vi "Build copy.vi"() -> ()   [LabVIEW 2017]
panel:
  out "Boolean Round":bool
  in  "stop":bool
  in  "Copy":bool
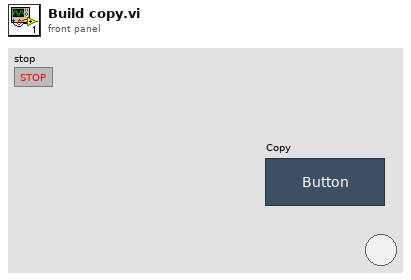
[diagram p1: front panel]
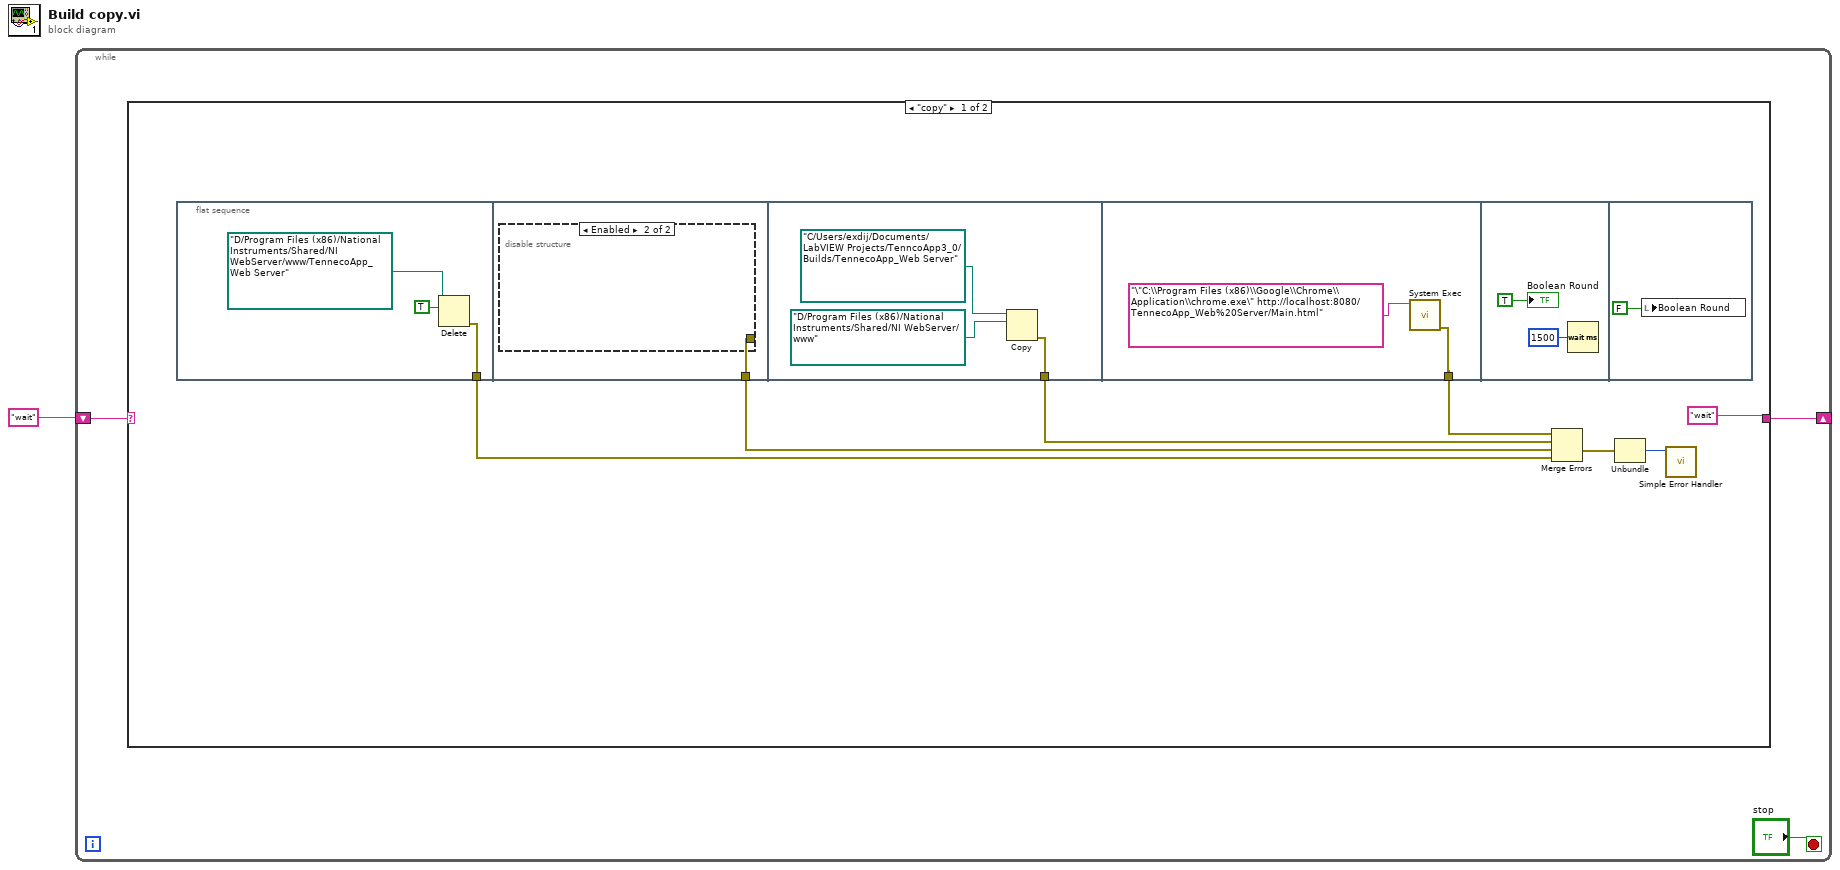
[diagram p0: block diagram]
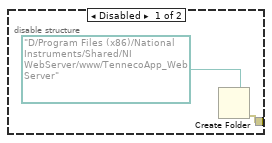
[diagram p2: hidden frame]
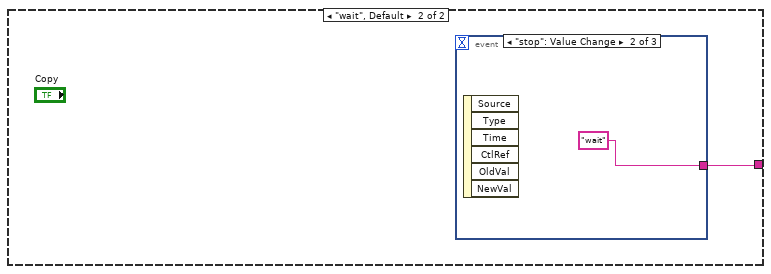
[diagram p3: hidden frame]
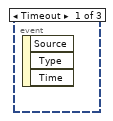
[diagram p4: hidden frame]
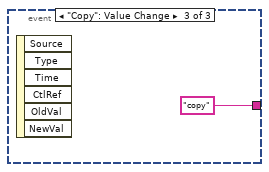
[diagram p5: hidden frame]
diagram:
  n1 = while {
    shift-right: [w3] -> _
    shift-left: "wait" -> [w4]
    stop <- "stop" stop-if-true
    n2 = case shown="\"copy\"" w4 {
      tunnel: ["wait" w26] -> w3
      frame "copy" {
        n3 = flat-sequence {
          tunnel: [w12] -> w10
          tunnel: [w15] -> w11
          tunnel: [w18] -> w6
          tunnel: [w21] -> w7
          frame #0 {
            n4 = Delete(path (use dialog)=path "D:/Program Files (x86)/National Instruments/Shared/NI WebServer/www/TennecoApp_Web Server" ("target path (use dialog)"), entire hierarchy (F)=TRUE) -> (error out=w12:errorcluster)  [unwired: 3 in, 2 out]
          }
          frame #1 {
            n5 = disable-structure shown="Enabled" {
              disable-tunnel: [w16 _] -> w15
              frame Disabled {
                n6 = Create Folder(path (use dialog)=path "D:/Program Files (x86)/National Instruments/Shared/NI WebServer/www/TennecoApp_Web Server" ("target path (use dialog)")) -> (error out=w16:errorcluster)  [unwired: 2 in, 2 out]
              }
              frame Enabled {
              }
            }
          }
          frame #2 {
            n7 = Copy(10:path "D:/Program Files (x86)/National Instruments/Shared/NI WebServer/www" ("target path (use dialog)"), 11:path "C:/Users/exdij/Documents/LabVIEW Projects/TenncoApp3_0/Builds/TennecoApp_Web Server" ("source path")) -> (0:w18:errorcluster)  [unwired: 3 in, 2 out]
          }
          frame #3 {
            n8 = call <vilib>:"System Exec.vi"("command line"="\"C:\\Program Files (x86)\\Google\\Chrome\\Application\\chrome.exe\" http://localhost:8080/TennecoApp_Web%20Server/Main.html") -> ("error out"=w21:errorcluster)  [unwired: 7 in, 3 out]
          }
          frame #4 {
            n9 = Wait (ms)(milliseconds to wait=u32 1500) -> ()  [unwired: 1 out]
            "Boolean Round" <- TRUE
          }
          frame #5 {
            n10 = local write "Boolean Round"(FALSE) -> ()
          }
        }
        n11 = Merge Errors(w7, w6, w11, w10) -> (w9:errorcluster)
        n12 = Unbundle(w9) -> ("code"=w8:i32)  [unwired: 2 out]
        n13 = call <vilib>:"Simple Error Handler.vi"("error code (no error:0)"=w8) -> ()  [unwired: 4 in, 5 out]
      }
      frame "wait", Default {
        n14 = event shown="[1] \"stop\": Value Change" {
          selector: _ -> [_ _ _]
          dyn-events: _ -> [_ _ _]
          timeout: _ -> [_ _ _]
          tunnel: [_ "wait" "copy"] -> w26
          event Timeout {
            n15 = event-data() -> ()  [unwired: 1 in, 3 out]
          }
          event "stop": Value Change {
            n16 = event-data() -> ()  [unwired: 1 in, 6 out]
          }
          event "Copy": Value Change {
            n17 = event-data() -> ()  [unwired: 1 in, 6 out]
          }
        }
      }
    }
  }
